vi "Initialize.vi"(8 "error in (no error)":errorcluster, 11 "Modbus master in":refnum<class "Modbus Master.lvclass">) -> (0 "error out":errorcluster, 3 "Modbus master out":refnum<class "Modbus Master.lvclass">)   [LabVIEW 2020, in "Modbus Master.lvclass"]
doc: "Initializes a Modbus master instance. If using the <B>Create Modbus Instance</B> VI, this is not necessary. This function will initiate any required bus communication."
uses:
  <vilib>/Modbus/master/Modbus Master.lvclass
  <vilib>/Modbus/master/Modbus Master.lvclass/Modbus Master.ctl
  <vilib>/Modbus/subvis/Protocol/Interfaces/Network Master/Network Master.lvclass
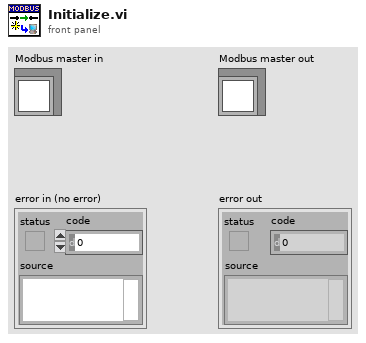
[diagram p1: front panel]
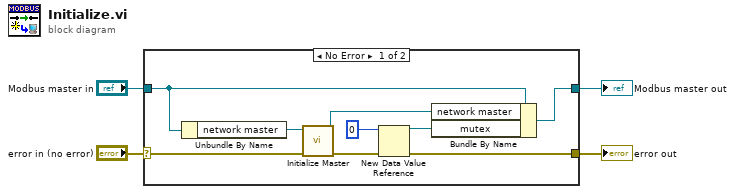
[diagram p0: block diagram]
diagram:
  n1 = case shown="No Error" "error in (no error)" {
    selector: "error in (no error)" -> [w5 w14]
    tunnel: [w13 w15] -> w4
    tunnel: "Modbus master in" -> [w11 w15]
    tunnel: [w8 w14] -> w2
    frame No Error {
      n2 = Unbundle By Name(w11) -> ("network master"=w10:refnum<class "Network Master.lvclass">)
      n3 = call-dynamic "Initialize Master.vi"("error in (no error)"=w5, "network master in"=w10) -> ("error out"=w9:errorcluster, "network master out"=w12:refnum<class "Network Master.lvclass">)  [unwired: 8 in]
      n4 = New Data Value Reference(data value=u8 0, error in=w9) -> (data value reference=w7:refnum<data-value>, error out=w8:errorcluster)
      n5 = Bundle By Name(cluster=w11, "network master"=w12, "mutex"=w7) -> (w13:refnum<class "Modbus Master.lvclass">)
    }
    frame Error {
    }
  }
  "error out" <- w2
  "Modbus master out" <- w4
